vi "Test Read Function Blocks.vi"(11 "TwinCAT ADS in":refnum<class "TwinCAT ADS.lvclass">) -> (3 "TwinCAT ADS out":refnum<class "TwinCAT ADS.lvclass">)   [LabVIEW 2018]
uses:
  TwinCAT ADS Class/TwinCAT ADS.lvclass
  Controls/FB_Simple.ctl
  Controls/FB_Packed.ctl
  Controls/FB_Complex.ctl
  Controls/ST_Complex.ctl
  Controls/Enum.ctl
  Controls/ST_Simple.ctl
  Controls/ST_Packed.ctl
  0f192603-4b3d-4f37-814b-8045268a4184.vi
  67a72bd1-5191-48bf-9b9a-0a1df22764e4.vi
  c8f2f14a-791d-4484-b25b-25e31bed0e1d.vi
  0e82c4fa-873b-4361-ac99-2e6e4b7cd392.vi
  da0f88be-82f8-4e5b-86e7-5baa69d9b51e.vi
  4782b519-43e7-4b8e-bd72-e209be860882.vi
  e7a7b24b-aede-49d7-b369-bb451e1de87e.vi
  TwinCAT ADS Class/VIs/Data/Read.vi
  <vilib>/addons/_JKI Toolkits/Caraya/classes/Assert/Assert True.vi
  <vilib>/addons/_JKI Toolkits/Caraya/classes/Assert/Assert.lvclass
  <vilib>/addons/_JKI Toolkits/Caraya/classes/Test/Test.lvclass
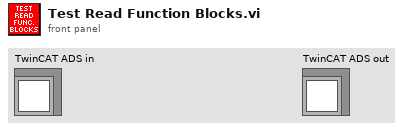
[diagram p1: front panel]
types:
  T1 = typedef "FB_Packed.ctl" = cluster{"bMember":bool, "nMember":i32, "sMember":string}
  T2 = typedef "FB_Complex.ctl" = cluster{"_fMember":dbl, "_stMember":T3, "_fbSimpleMember":T7, "_fbPackedMember":T1}
  T3 = typedef "ST_Complex.ctl" = cluster{"bMember":bool, "eMember":T4, "stSimpleMember":T5, "stPackedMember":T6, "FB_Simple":T7, "arrfMember":dbl[]}
  T4 = typedef "Enum.ctl" = enum16{"Member 0", "Member 1", "Member 2"}
  T5 = typedef "ST_Simple.ctl" = cluster{"bMember":bool, "dtMember":timestamp, "nMember":i32}
  T6 = typedef "ST_Packed.ctl" = cluster{"bMember":bool, "dtMember":timestamp, "fMember":dbl}
  T7 = typedef "FB_Simple.ctl" = cluster{"_bMember":bool, "_nMember":i32, "_sMember":string}
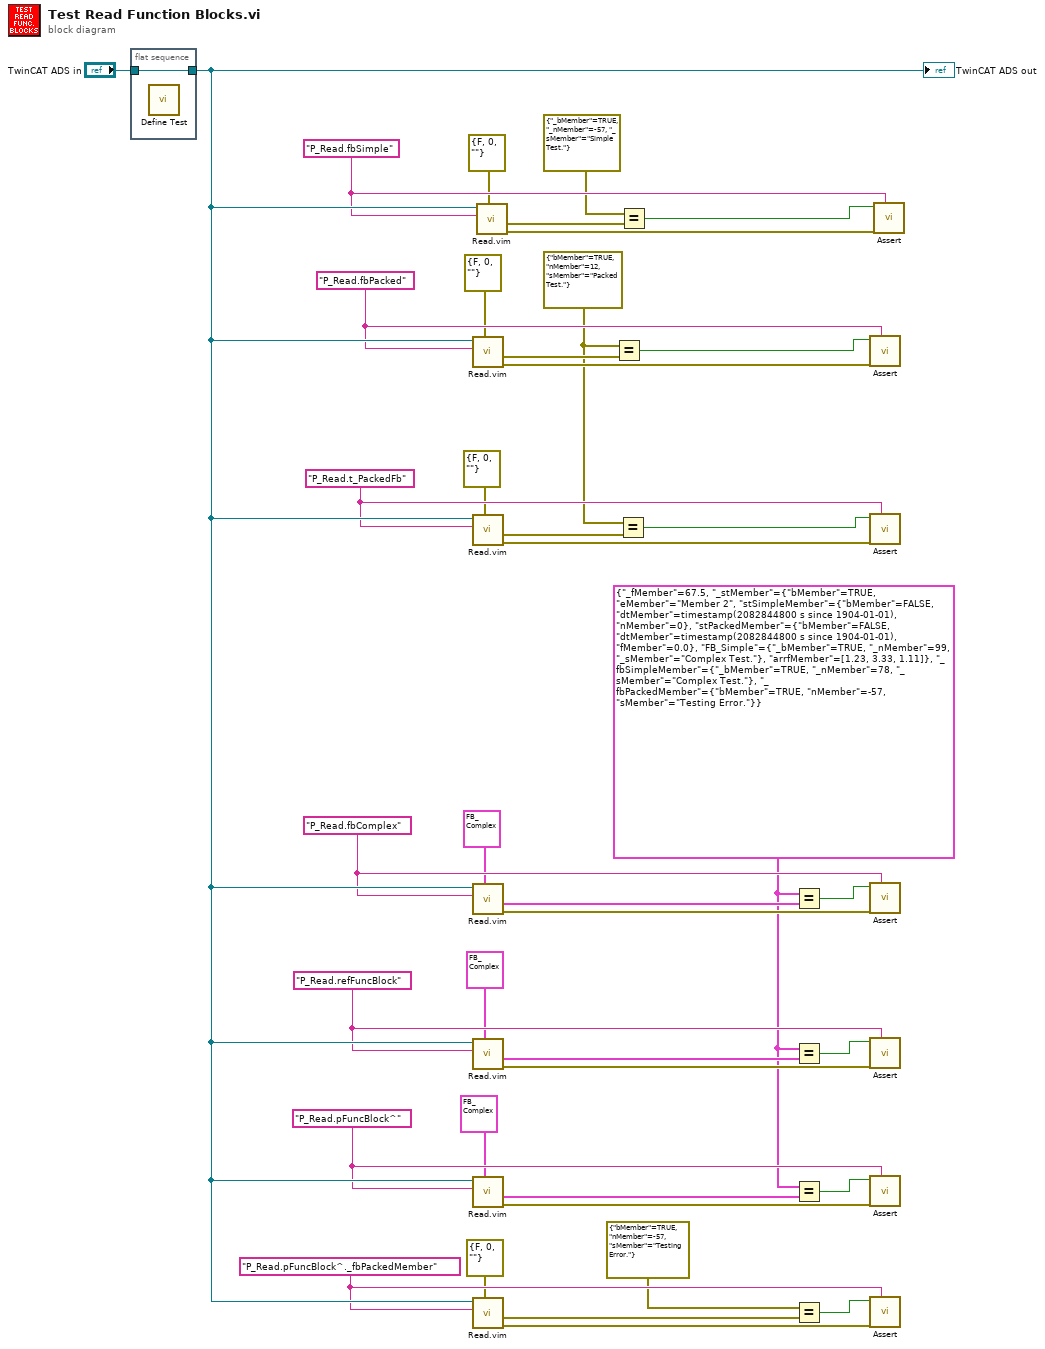
[diagram p0: block diagram]
diagram:
  w3 = T2 {"_fMember"=67.5, "_stMember"={"bMember"=TRUE, "eMember"=enum."Member 2", "stSimpleMember"={"bMember"=FALSE, "dtMember"=timestamp(2082844800 s since 1904-01-01), "nMember"=0}, "stPackedMember"={"bMember"=FALSE, "dtMember"=timestamp(2082844800 s since 1904-01-01), "fMember"=0.0}, "FB_Simple"={"_bMember"=TRUE, "_nMember"=99, "_sMember"="Complex Test."}, "arrfMember"=[1.23, 3.33, 1.11]}, "_fbSimpleMember"={"_bMember"=TRUE, "_nMember"=78, "_sMember"="Complex Test."}, "_fbPackedMember"={"bMember"=TRUE, "nMember"=-57, "sMember"="Testing Error."}} ("Value")
  w8 = T1 {"bMember"=TRUE, "nMember"=12, "sMember"="Packed Test."} ("FB_Packed")
  w13 = "P_Read.pFuncBlock^._fbPackedMember" ("Symbol Name")
  w20 = "P_Read.pFuncBlock^" ("Symbol Name")
  w21 = "P_Read.refFuncBlock" ("Symbol Name")
  w33 = "P_Read.fbComplex" ("Symbol Name")
  w34 = "P_Read.t_PackedFb" ("Symbol Name")
  w37 = "P_Read.fbPacked" ("Symbol Name")
  w38 = "P_Read.fbSimple" ("Symbol Name")
  n1 = flat-sequence {
    tunnel: "TwinCAT ADS in" -> [w42]
    tunnel: [w42] -> w41
    frame #0 {
      n2 = call <vilib>:"Define Test.vi"() -> ()  [unwired: 10 in, 2 out]
    }
  }
  n3 = call "Read.vim"("Type"=T1 {"bMember"=FALSE, "nMember"=0, "sMember"=""} ("FB_Packed"), "Symbol Name"=w37, "TwinCAT ADS in"=w41) -> ("error out"=w36:errorcluster, "Value"=w29:T1)  [unwired: 6 in, 1 out]
  n4 = call "Read.vim"("Type"=T1 {"bMember"=FALSE, "nMember"=0, "sMember"=""} ("FB_Packed"), "Symbol Name"=w34, "TwinCAT ADS in"=w41) -> ("error out"=w35:errorcluster, "Value"=w27:T1)  [unwired: 6 in, 1 out]
  n5 = call "Read.vim"("Type"=T2 {"_fMember"=0.0, "_stMember"={"bMember"=FALSE, "eMember"=enum."Member 0", "stSimpleMember"={"bMember"=FALSE, "dtMember"=timestamp(0 s since 1904-01-01), "nMember"=0}, "stPackedMember"={"bMember"=FALSE, "dtMember"=timestamp(0 s since 1904-01-01), "fMember"=0.0}, "FB_Simple"={"_bMember"=FALSE, "_nMember"=0, "_sMember"=""}, "arrfMember"=[]}, "_fbSimpleMember"={"_bMember"=FALSE, "_nMember"=0, "_sMember"=""}, "_fbPackedMember"={"bMember"=FALSE, "nMember"=0, "sMember"=""}} ("FB_Complex"), "Symbol Name"=w33, "TwinCAT ADS in"=w41) -> ("error out"=w32:errorcluster, "Value"=w4:T2)  [unwired: 6 in, 1 out]
  n6 = call "Read.vim"("Type"=T2 {"_fMember"=0.0, "_stMember"={"bMember"=FALSE, "eMember"=enum."Member 0", "stSimpleMember"={"bMember"=FALSE, "dtMember"=timestamp(0 s since 1904-01-01), "nMember"=0}, "stPackedMember"={"bMember"=FALSE, "dtMember"=timestamp(0 s since 1904-01-01), "fMember"=0.0}, "FB_Simple"={"_bMember"=FALSE, "_nMember"=0, "_sMember"=""}, "arrfMember"=[]}, "_fbSimpleMember"={"_bMember"=FALSE, "_nMember"=0, "_sMember"=""}, "_fbPackedMember"={"bMember"=FALSE, "nMember"=0, "sMember"=""}} ("FB_Complex"), "Symbol Name"=w21, "TwinCAT ADS in"=w41) -> ("error out"=w22:errorcluster, "Value"=w23:T2)  [unwired: 6 in, 1 out]
  n7 = call "Read.vim"("Type"=T2 {"_fMember"=0.0, "_stMember"={"bMember"=FALSE, "eMember"=enum."Member 0", "stSimpleMember"={"bMember"=FALSE, "dtMember"=timestamp(0 s since 1904-01-01), "nMember"=0}, "stPackedMember"={"bMember"=FALSE, "dtMember"=timestamp(0 s since 1904-01-01), "fMember"=0.0}, "FB_Simple"={"_bMember"=FALSE, "_nMember"=0, "_sMember"=""}, "arrfMember"=[]}, "_fbSimpleMember"={"_bMember"=FALSE, "_nMember"=0, "_sMember"=""}, "_fbPackedMember"={"bMember"=FALSE, "nMember"=0, "sMember"=""}} ("FB_Complex"), "Symbol Name"=w20, "TwinCAT ADS in"=w41) -> ("error out"=w19:errorcluster, "Value"=w18:T2)  [unwired: 6 in, 1 out]
  n8 = call "Read.vim"("Type"=T1 {"bMember"=FALSE, "nMember"=0, "sMember"=""} ("FB_Packed"), "Symbol Name"=w13, "TwinCAT ADS in"=w41) -> ("error out"=w14:errorcluster, "Value"=w15:T1)  [unwired: 6 in, 1 out]
  n9 = call "Read.vim"("Type"=T7 {"_bMember"=FALSE, "_nMember"=0, "_sMember"=""} ("FB_Simple"), "Symbol Name"=w38, "TwinCAT ADS in"=w41) -> ("error out"=w40:errorcluster, "Value"=w31:T7)  [unwired: 6 in, 1 out]
  n10 = Equal?(x=w8, y=w29) -> (x = y?=w28:bool)
  n11 = Equal?(x=w8, y=w27) -> (x = y?=w26:bool)
  n12 = Equal?(x=T7 {"_bMember"=TRUE, "_nMember"=-57, "_sMember"="Simple Test."} ("FB_Simple"), y=w31) -> (x = y?=w30:bool)
  n13 = Equal?(x=w3, y=w4) -> (x = y?=w25:bool)
  n14 = Equal?(x=w3, y=w23) -> (x = y?=w24:bool)
  n15 = Equal?(x=w3, y=w18) -> (x = y?=w17:bool)
  n16 = Equal?(x=T1 {"bMember"=TRUE, "nMember"=-57, "sMember"="Testing Error."} ("_fbPackedMember"), y=w15) -> (x = y?=w16:bool)
  n17 = call-poly <vilib>:"Assert.vi"("Label"=w37, "error in (no error)"=w36, "True?"=w28) -> ()  [unwired: 7 in, 2 out]
  n18 = call-poly <vilib>:"Assert.vi"("Label"=w34, "error in (no error)"=w35, "True?"=w26) -> ()  [unwired: 7 in, 2 out]
  n19 = call-poly <vilib>:"Assert.vi"("Label"=w33, "error in (no error)"=w32, "True?"=w25) -> ()  [unwired: 7 in, 2 out]
  n20 = call-poly <vilib>:"Assert.vi"("Label"=w21, "error in (no error)"=w22, "True?"=w24) -> ()  [unwired: 7 in, 2 out]
  n21 = call-poly <vilib>:"Assert.vi"("Label"=w20, "error in (no error)"=w19, "True?"=w17) -> ()  [unwired: 7 in, 2 out]
  n22 = call-poly <vilib>:"Assert.vi"("Label"=w13, "error in (no error)"=w14, "True?"=w16) -> ()  [unwired: 7 in, 2 out]
  n23 = call-poly <vilib>:"Assert.vi"("Label"=w38, "error in (no error)"=w40, "True?"=w30) -> ()  [unwired: 7 in, 2 out]
  "TwinCAT ADS out" <- w41
